vi "Entry.vi"(8 "error in (no error)":errorcluster, 11 "New State":refnum<class "Command States.lvclass">) -> (0 "error out":errorcluster, 3 "State out":refnum<class "Command States.lvclass">)   [LabVIEW 2013, in "Command Actor.lvlib" / "Command States.lvclass"]
doc: "This is an abstract method. Override this method to define the behavior when you enter the state."
uses:
  Command States.lvclass
  <vilib>/ni/Actors/State Actor/State Actor/State Actor.lvclass
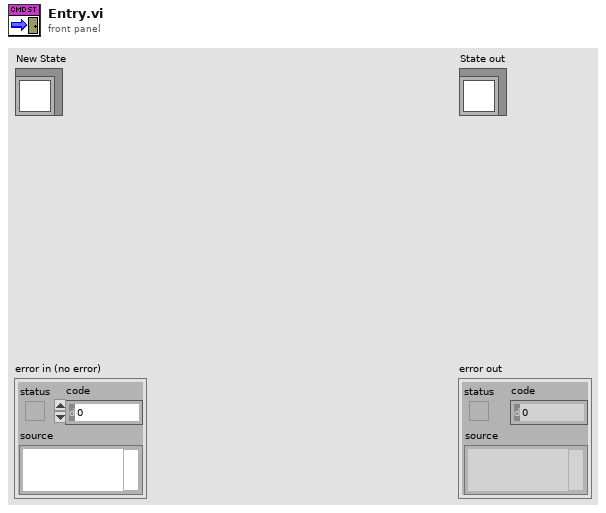
[diagram p1: front panel]
types:
  T1 = typedef "Command Actor.lvlib/Command States.lvclass/State Status.ctl" = cluster{"State Name":string, "State Entry Time":timestamp, "State Exit Time":timestamp}
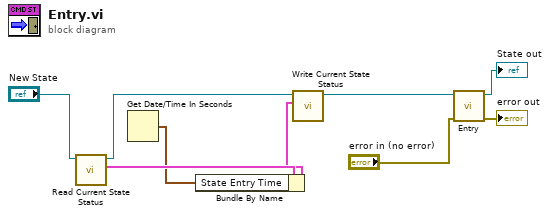
[diagram p0: block diagram]
diagram:
  n1 = call-dynamic "Read Current State Status.vi"("Command States in"="New State") -> ("State Status"=w3:T1, "Command States out"=w4:refnum<class "Command States.lvclass">)  [unwired: 8 in, 1 out]
  n2 = Get Date/Time In Seconds() -> (seconds since 1Jan1904=w1:timestamp)
  n3 = Bundle By Name(cluster=w3, "State Entry Time"=w1) -> (w2:T1)
  n4 = call-dynamic "Write Current State Status.vi"("State Status"=w2, "Command States in"=w4) -> ("Command States out"=w6:refnum<class "Command States.lvclass">)  [unwired: 8 in, 1 out]
  n5 = call-parent "Entry.vi"("error in (no error)"="error in (no error)", "New State"=w6) -> ("error out"=→"error out":errorcluster, "State out"=→"State out":refnum<class "Command States.lvclass">)  [unwired: 8 in]
